vi "step-force-map.vi"() -> ()   [LabVIEW 2017]
uses:
  controls/boolean_info.ctl
  sysID_Z-axis-params.ctl
  <vilib>/rvi/Emulation/niFpgaGetClockAttributes.vi
  <vilib>/rvi/Emulation/niFpgaSctlEmulationGetInTimedLoop.vi
  <vilib>/rvi/Emulation/niFpgaEmulationReportErrorSimple.vi
  <vilib>/rvi/Emulation/niFpgaProcessEmulError.vi
  <vilib>/rvi/eio/common/nirviEmuTemplateMethod_errors.vi
  <vilib>/rvi/Emulation/niFpgaEmulationIsFPGAContextNoSignature.vi
  <vilib>/rvi/DataTransferAndStorage/Container/Common/niFpgaContainerGetUniqueNameForEmu.vi
  <vilib>/rvi/Memory/Memory_Emulation/niFpgaMemoryEmulationCacheClearOnFirstRun.vi
  <vilib>/rvi/Memory/Memory_Emulation/nirvimemoryEmulationManagerCache_MakeExclusive.vi
  <vilib>/rvi/Memory/Memory_Emulation/niFpgaMemoryEmulationValidateCache.vi
  <vilib>/rvi/Memory/Memory_Emulation/nirvimemoryEmulationManagerCache_InsertValue.vi
  <vilib>/Utility/error.llb/Clear Errors.vi
  <vilib>/rvi/Memory/Memory_Emulation/nirvimemoryEmulationManagerCache_ReleaseExclusive.vi
  <vilib>/rvi/Memory/Memory_Emulation/nirvimemoryEmulationManagerCache_GetValue.vi
  <vilib>/rvi/Memory/Memory_Emulation/nirvimemoryEmulationManagerCache_SetValue.vi
  <vilib>/rvi/Emulation/niFpgaCriticalErrorInLSC.vi
  <vilib>/eio/EIONode/EIONode.xnode
  <vilib>/rvi/DataTransferAndStorage/Container/XNode/niFpgaContainer.xnode
  <vilib>/rvi/DataTransferAndStorage/Register/Emulation/niFpgaRegisterEmulation.vi
  libimaging-cs.lvlib
panel:
  in  "N-UP":i16
  in  "Z-up":sgl format="%#_13g"
  in  "z-down-max":fxp<+/-,32,16>
  out "logging-timeout?":bool
  in  "sysID_Z_axis_params":T1={"TOL"=0.3, "ramp-rate"=-5e-06, "z-u-max"=5.0, "offset"=0.0, "Ki"=0.001, "Z-error-threshold"=0.0, "Z-settled-samples\nthreshold "=0, "z_UP"=1.5, "zup-N"=5000} {"Z-error-threshold" format="%#_13g"; "ramp-rate" format="%#_4g"; "TOL" format="%#_13g"}
  out "iter":i32
  out "All Done":bool
  in  "TsTicks":u32=1600
  out "Current Case":i16
  out "boolean \nindicators":T2
  out "z-u(k)":sgl
  in  "ABORT":bool
  out "e(0) (threshhold init)":fxp<+/-,16,5>
  in  "init Z up":fxp<+/-,16,5>
  in  "trigger-0":bool
  in  "initial case":i16
  # "- If collect all = fasle and collect move = false,\nwe only collect measurement data.\n- If collect all = false, and collect move = true,\nwe collect measurement and move data.\n- If collect all = true, we collect everything."
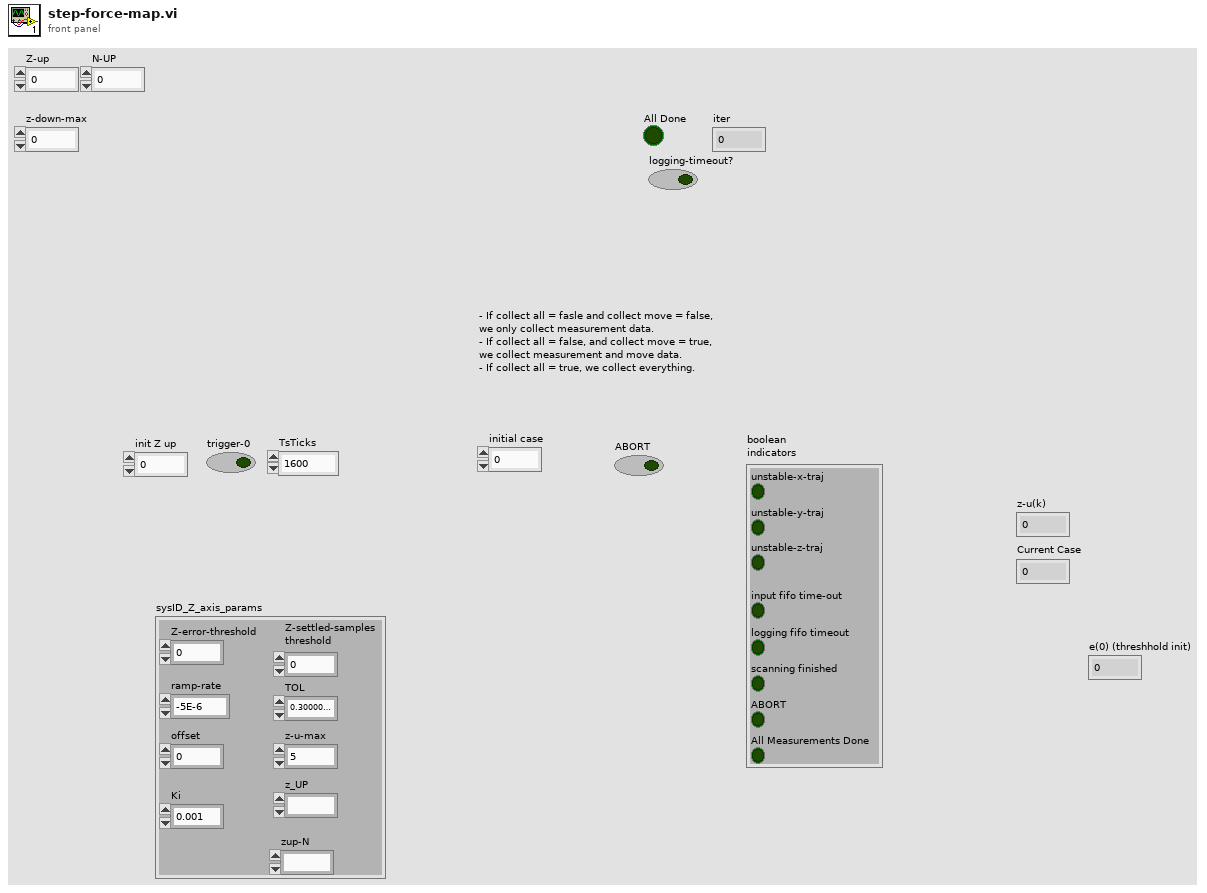
[diagram p1: front panel]
types:
  T1 = typedef "sysID_Z-axis-params.ctl" = cluster{"TOL":sgl, "ramp-rate":sgl, "z-u-max":sgl, "offset":sgl, "Ki":sgl, "Z-error-threshold":sgl, "Z-settled-samples\nthreshold ":i16, "z_UP":fxp<+/-,16,5>, "zup-N":i16}
  T2 = typedef "boolean_info.ctl" = cluster{"unstable-z-traj":bool, "input fifo time-out":bool, "logging fifo timeout":bool, "scanning finished":bool, "unstable-x-traj":bool, "unstable-y-traj":bool, "ABORT":bool, "All Measurements Done":bool}
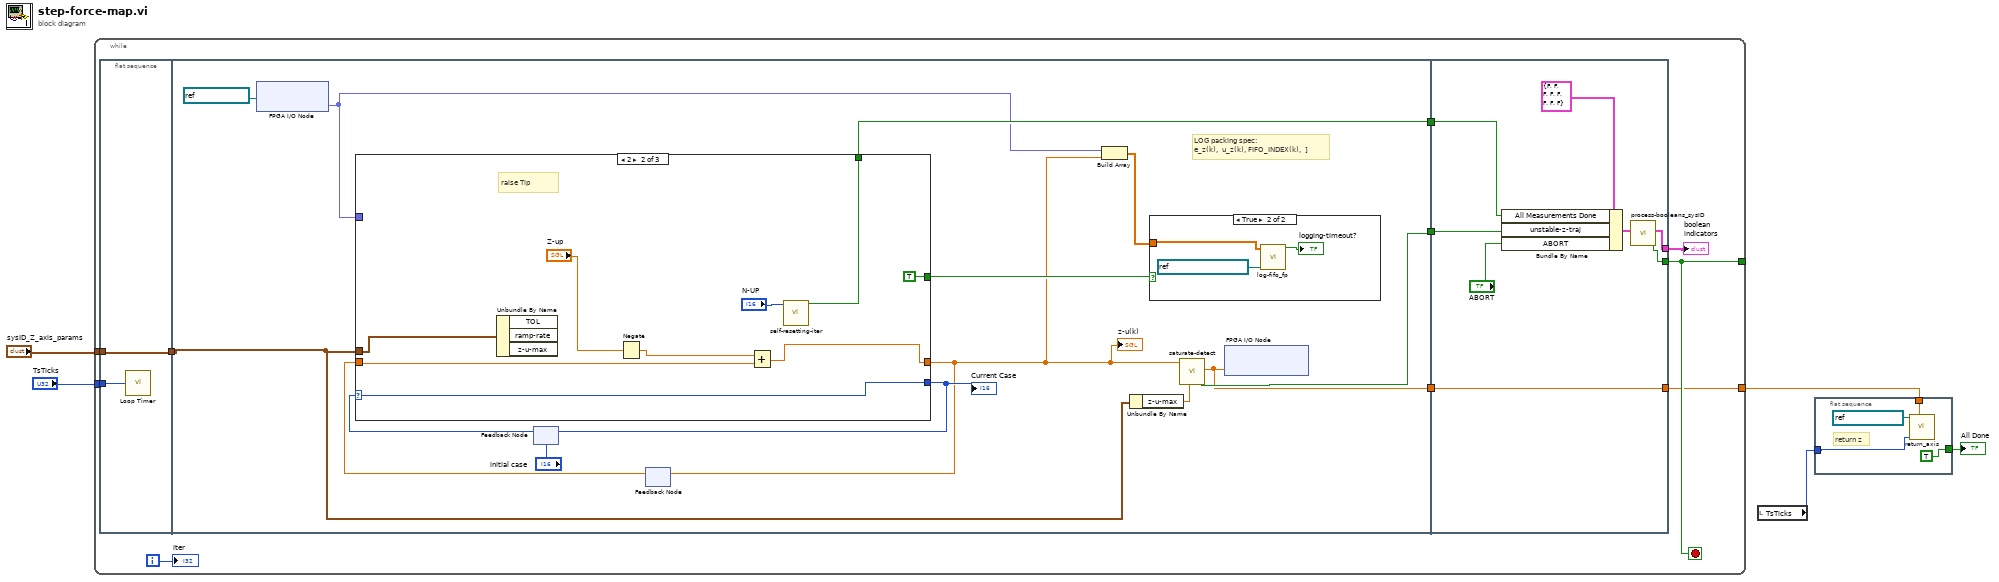
[diagram p0: block diagram]
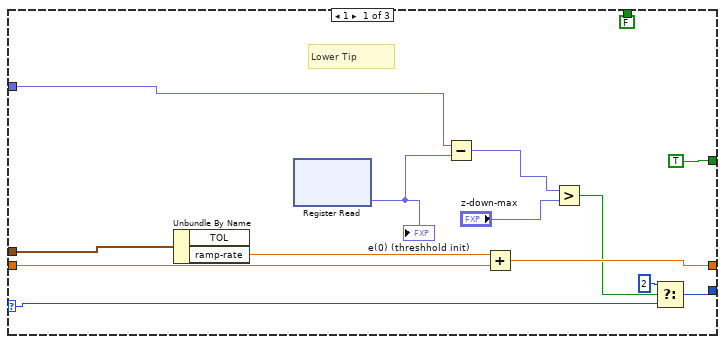
[diagram p3: hidden frame]
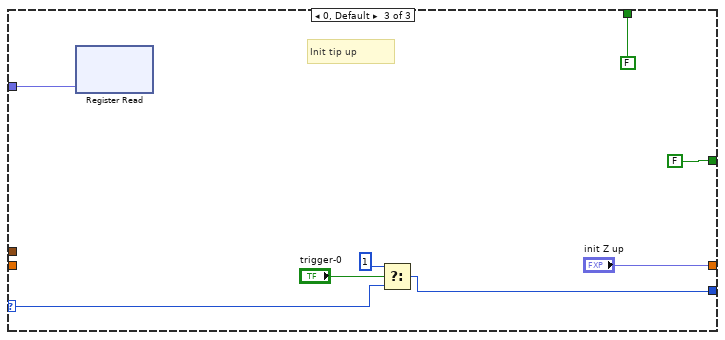
[diagram p4: hidden frame]
diagram:
  n1 = while {
    tunnel: "sysID_Z_axis_params" -> [w12]
    tunnel: "TsTicks" -> [w11]
    tunnel: [w9] -> _
    tunnel: [w7] -> w4
    i -> [w6]
    stop <- w9 stop-if-true
    n2 = flat-sequence {
      tunnel: w11 -> [w16]
      tunnel: w12 -> [w17]
      tunnel: [w17] -> w15
      tunnel: w15 -> [w25]
      tunnel: [w27] -> w14
      tunnel: [w23] -> w13
      tunnel: [w26] -> w8
      tunnel: w14 -> [w73]
      tunnel: w13 -> [w70]
      tunnel: [w66] -> w9
      tunnel: [w67] -> w10
      tunnel: [w69] -> w7
      tunnel: w8 -> [w69]
      frame #0 {
        n3 = call "Loop Timer"("Count(Ticks)"=w16) -> ()  [unwired: 1 out]
      }
      frame #1 {
        # "LOG packing spec:\ne_z(k),  u_z(k), FIFO_INDEX(k),  ]"
        n4 = xnode "FPGA I/O Node"("FPGA I/O In"=refnum<k21> "Mod2/AI2" ("y - ADC")) -> ("I/O Item"=w19:fxp<+/-,24,5>)  [unwired: 1 out]
        n5 = feedback #1("initial case") -> (w30:i16)
        n6 = feedback #2() -> (w29:sgl)  [unwired: 1 in]
        n7 = case shown="2" w30 {
          selector: w30 -> [w47 w57 w63]
          tunnel: [TRUE TRUE ("trigger-0") FALSE] -> w21
          tunnel: [w45 w57 w65] -> w22
          tunnel: w19 -> [w37 _ w59]
          tunnel: [w40 w53 "init Z up"] -> w18
          tunnel: w29 -> [w43 w55 _]
          tunnel: w25 -> [w46 w56 _]
          tunnel: [FALSE w50 FALSE] -> w23
          frame 1 {
            # "Lower Tip"
            n8 = Unbundle By Name(w46) -> ("ramp-rate"=w48:sgl)  [unwired: 1 out]
            n9 = xnode ("Register Read")() -> ("Data"=w36:fxp<+/-,16,5>)  [unwired: 1 in, 1 out]
            "e(0) (threshhold init)" <- w36
            n10 = Subtract(x=w37, y=w36) -> (x-y=w35:fxp<+/-,25,6>)
            n11 = Add(x=w48, y=w43) -> (x+y=w40:sgl)
            n12 = Greater?(x=w35, y="z-down-max") -> (0:w38:bool)
            n13 = Select(t=i16 2, s=w38, f=w47) -> (s? t:f=w45:i16)
          }
          frame 2 {
            # "raise Tip"
            n14 = Unbundle By Name(w56) -> ()  [unwired: 3 out]
            n15 = Negate(x="Z-up") -> (-x=w54:sgl)
            n16 = Add(x=w54, y=w55) -> (x+y=w53:sgl)
            n17 = call "self-resetting-iter.vi"("N"="N-UP") -> ("Boolean"=w50:bool)  [unwired: 9 in, 1 out]
          }
          frame 0, Default {
            # "Init tip up"
            n18 = xnode ("Register Read")("Data"=w59) -> ()  [unwired: 1 in, 1 out]
            n19 = Select(t=i16 1, s="trigger-0", f=w63) -> (s? t:f=w65:i16)
          }
        }
        "z-u(k)" <- w18
        "Current Case" <- w22
        n20 = feedback-in #1(w22) -> ()
        n21 = feedback-in #2(w18) -> ()
        n22 = Build Array(w19, w18) -> (w28:sgl[])
        n23 = Unbundle By Name(w25) -> ("z-u-max"=w24:sgl)
        n24 = case shown="True" w21 {
          tunnel: w28 -> [_ w34]
          frame False {
          }
          frame True {
            n25 = call "log-fifo_fp.vi"("FIFO In"=refnum<k21> "fpga_to_host_fp", "input-data"=w34) -> ("logging-timeout?"=→"logging-timeout?":bool)  [unwired: 9 in]
          }
        }
        n26 = call "saturate-detect.vi"("bound"=w24, "x"=w18) -> ("saturated"=w27:bool, "sat(x)"=w26:sgl)  [unwired: 8 in]
        n27 = xnode "FPGA I/O Node"("Mod1/AO2"=w26) -> ()  [unwired: 1 in, 1 out]
      }
      frame #2 {
        n28 = Bundle By Name(cluster=T2 {"unstable-z-traj"=FALSE, "input fifo time-out"=FALSE, "logging fifo timeout"=FALSE, "scanning finished"=FALSE, "unstable-x-traj"=FALSE, "unstable-y-traj"=FALSE, "ABORT"=FALSE, "All Measurements Done"=FALSE} ("boolean errors"), "All Measurements Done"=w70, "unstable-z-traj"=w73, "ABORT"="ABORT") -> (w68:T2)
        n29 = call "process-booleans_sysID.vi"("boolean indicators 2"=w68) -> ("scaning finished"=w66:bool, "boolean indicators"=w67:T2)  [unwired: 9 in]
      }
    }
    "boolean \nindicators" <- w10
    "iter" <- w6
  }
  n30 = local read "TsTicks"() -> (w1:u32)
  n31 = flat-sequence {
    tunnel: w4 -> [w77]
    tunnel: [TRUE] -> w3
    tunnel: w1 -> [w74]
    frame #0 {
      # "return z"
      n32 = call "return_axis.vi"("u(0)"=w77, "TsTicks"=w74, "FPGA I/O In"=refnum<k21> "Mod1/AO2") -> ()  [unwired: 9 in]
    }
  }
  "All Done" <- w3
